vi "Set Property Type.vi"(8 "error in":errorcluster, 11 "Property Node":refnum<k20>) -> (0 "error out":errorcluster, 2 "Property Type":T1, 3 "Property Type Node":refnum<k20>)   [LabVIEW 2024, in "Config File Parser.lvlib" / "Property.lvclass"]
uses:
  Property.lvclass
  Property Type.ctl
  <vilib>/xml/Close Reference(Node).vi
  Property.lvclass/Property.ctl
  <vilib>/xml/NI_XML.lvlib
  <resource>/objmgr/DOMUserDefRef.rc
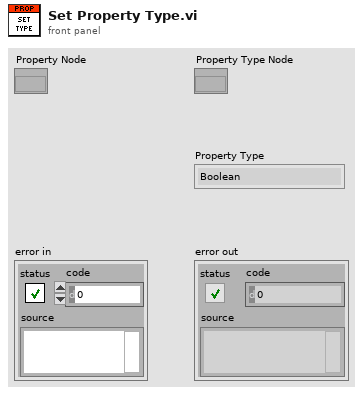
[diagram p1: front panel]
types:
  T1 = typedef "Config File Parser.lvlib/Property.lvclass/Property Type.ctl" = enum16{"Boolean", "Double", "String", "Path", "Dictionary", "DependentFile", "I16", "I32", "I64", "U16", "U32", "U64", "BooleanArray", "DoubleArray", "StringArray", "I16Array", "I32Array", "I64Array", "U16Array", "U32Array", "U64Array", "Variant"}
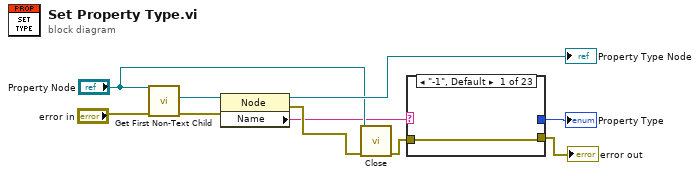
[diagram p0: block diagram]
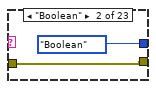
[diagram p2: hidden frame]
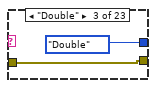
[diagram p3: hidden frame]
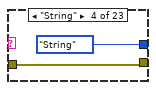
[diagram p4: hidden frame]
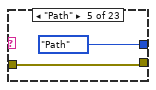
[diagram p5: hidden frame]
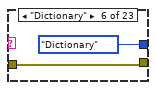
[diagram p6: hidden frame]
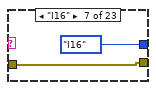
[diagram p7: hidden frame]
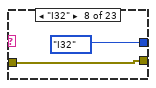
[diagram p8: hidden frame]
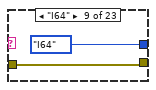
[diagram p9: hidden frame]
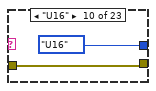
[diagram p10: hidden frame]
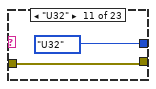
[diagram p11: hidden frame]
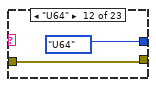
[diagram p12: hidden frame]
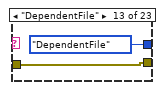
[diagram p13: hidden frame]
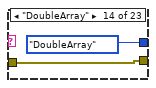
[diagram p14: hidden frame]
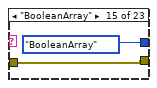
[diagram p15: hidden frame]
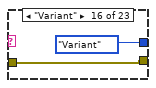
[diagram p16: hidden frame]
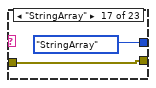
[diagram p17: hidden frame]
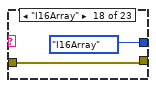
[diagram p18: hidden frame]
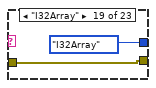
[diagram p19: hidden frame]
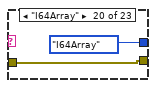
[diagram p20: hidden frame]
diagram:
  n1 = call <vilib>:"Get First Non-Text Child.vi"("error in (no error)"="error in", "node in"="Property Node") -> ("error out"=w9:errorcluster, "child node"=w5:refnum<k20>)  [unwired: 6 in, 2 out]
  n2 = property on="Property Node" class="Node"(reference=w5, error in=w9) -> (reference out=→"Property Type Node":refnum<k20>, error out=w8:errorcluster, "Name"=w2:string)
  n3 = call-poly <vilib>:"Close.vi"("error in (no error)"=w8, "node"="Property Node") -> ("error out"=w7:errorcluster)  [unwired: 7 in]
  n4 = case shown="\"-1\", Default" w2 {
    tunnel: [_ Property_Type."Boolean" ("Type") Property_Type."Double" ("Type") Property_Type."String" ("Type") Property_Type."Path" ("Type") Property_Type."Dictionary" ("Type") Property_Type."I16" ("Type") Property_Type."I32" ("Type") Property_Type."I64" ("Type") Property_Type."U16" ("Type") Property_Type."U32" ("Type") Property_Type."U64" ("Type") Property_Type."DependentFile" ("Type") Property_Type."DoubleArray" ("Type") Property_Type."BooleanArray" ("Type") Property_Type."Variant" ("Type") Property_Type."StringArray" ("Type") Property_Type."I16Array" ("Type") Property_Type."I32Array" ("Type") Property_Type."I64Array" ("Type") Property_Type."U16Array" ("Type") Property_Type."U32Array" ("Type") Property_Type."U64Array" ("Type")] -> w1
    tunnel: w7 -> [w11 w13 w15 w17 w19 w21 w23 w25 w27 w29 w31 w33 w35 w37 w39 w41 w43 w45 w47 w49 w51 w53 w55]
    tunnel: [w11 w13 w15 w17 w19 w21 w23 w25 w27 w29 w31 w33 w35 w37 w39 w41 w43 w45 w47 w49 w51 w53 w55] -> w6
    frame "-1", Default {
    }
    frame "Boolean" {
    }
    frame "Double" {
    }
    frame "String" {
    }
    frame "Path" {
    }
    frame "Dictionary" {
    }
    frame "I16" {
    }
    frame "I32" {
    }
    frame "I64" {
    }
    frame "U16" {
    }
    frame "U32" {
    }
    frame "U64" {
    }
    frame "DependentFile" {
    }
    frame "DoubleArray" {
    }
    frame "BooleanArray" {
    }
    frame "Variant" {
    }
    frame "StringArray" {
    }
    frame "I16Array" {
    }
    frame "I32Array" {
    }
    frame "I64Array" {
    }
    frame "U16Array" {
    }
    frame "U32Array" {
    }
    frame "U64Array" {
    }
  }
  "Property Type" <- w1
  "error out" <- w6
